vi "Draw Goals.vi"(11 "2D Picture":picture) -> (3 "2D Picture 2":picture)   [LabVIEW 2013]
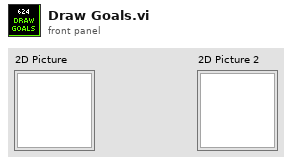
[diagram p1: front panel]
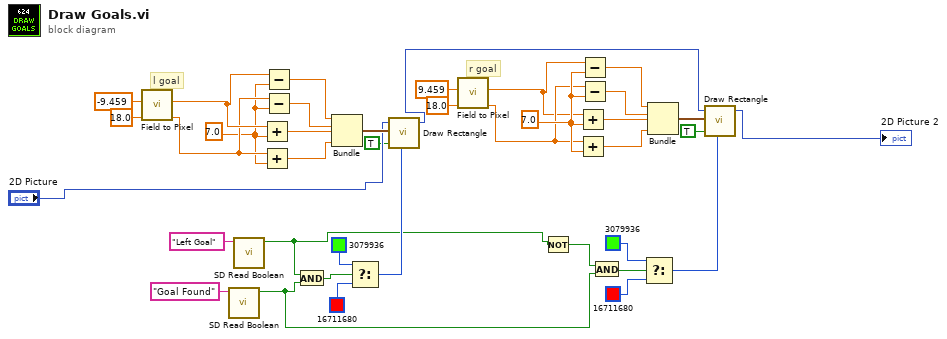
[diagram p0: block diagram]
diagram:
  w20 = 7.0
  w34 = 7.0
  # "r goal"
  # "l goal"
  n1 = call "Field to Pixel.vi"("Field Coordinate Y"=18.0, "Field Coordinate X"=-9.459) -> ("Pixel Y"=w35:dbl, "Pixel X"=w36:dbl)  [unwired: 8 in]
  n2 = call <vilib>:"SD Read Boolean.vi"("Name"="Goal Found") -> ("Boolean"=w5:bool)  [unwired: 8 in, 2 out]
  n3 = call <vilib>:"SD Read Boolean.vi"("Name"="Left Goal") -> ("Boolean"=w7:bool)  [unwired: 8 in, 2 out]
  n4 = Add(x=w36, y=w34) -> (x+y=w30:dbl)
  n5 = Add(x=w35, y=w34) -> (x+y=w29:dbl)
  n6 = Subtract(x=w36, y=w34) -> (x-y=w32:dbl)
  n7 = Subtract(x=w35, y=w34) -> (x-y=w31:dbl)
  n8 = And(x=w7, y=w5) -> (x .and. y?=w11:bool)
  n9 = Bundle(w32, w31, w30, w29) -> (w33:cluster{dbl, dbl, dbl, dbl})  [unwired: 1 in]
  n10 = Select(t=u32 3079936 ("color(black)"), s=w11, f=u32 16711680 ("color(black)")) -> (s? t:f=w8:u32)
  n11 = call <vilib>:"Draw Rectangle.vi"("picture"="2D Picture", "rect"=w33, "fill?(F)"=TRUE, "color(black)"=w8) -> ("new picture"=w15:picture)  [unwired: 5 in]
  n12 = call "Field to Pixel.vi"("Field Coordinate Y"=18.0, "Field Coordinate X"=9.459) -> ("Pixel Y"=w19:dbl, "Pixel X"=w18:dbl)  [unwired: 8 in]
  n13 = Not(x=w7) -> (.not. x?=w6:bool)
  n14 = Add(x=w18, y=w20) -> (x+y=w24:dbl)
  n15 = Add(x=w19, y=w20) -> (x+y=w25:dbl)
  n16 = Subtract(x=w18, y=w20) -> (x-y=w22:dbl)
  n17 = Subtract(x=w19, y=w20) -> (x-y=w23:dbl)
  n18 = And(x=w6, y=w5) -> (x .and. y?=w3:bool)
  n19 = Select(t=u32 3079936 ("color(black)"), s=w3, f=u32 16711680 ("color(black)")) -> (s? t:f=w1:u32)
  n20 = Bundle(w22, w23, w24, w25) -> (w21:cluster{dbl, dbl, dbl, dbl})  [unwired: 1 in]
  n21 = call <vilib>:"Draw Rectangle.vi"("picture"=w15, "rect"=w21, "fill?(F)"=TRUE, "color(black)"=w1) -> ("new picture"=→"2D Picture 2":picture)  [unwired: 5 in]
